vi "sensor de luz.vi"(8 "Error In":errorcluster, 10 "PIN Fotoresistencia":u8, 11 "LINX Resource":T1) -> (0 "Error Out":errorcluster, 2 "Miles de lumenes":dbl, 3 "LINX Resource 2":T1, 4 "Estado":string)   [LabVIEW 2014]
uses:
  <vilib>/MakerHub/LINX/Private/Type Defs/LINX Ref.ctl
  <vilib>/MakerHub/LINX/Private/Type Defs/Platform.ctl
  <vilib>/MakerHub/LINX/Private/Type Defs/Interface.ctl
  <vilib>/MakerHub/LINX/Private/Device/Type Defs/LINX Device Config.ctl
  <vilib>/MakerHub/LINX/Private/Device/Type Defs/TCP Config.ctl
  <vilib>/MakerHub/LINX/Private/Device/Type Defs/Channels.ctl
  <vilib>/MakerHub/LINX/Public/Peripherals/Analog/Analog Read 1 Chan.vi
  <vilib>/MakerHub/LINX/LMH-LINX.lvlib
  <vilib>/MakerHub/LINX/Private/Device/Device.lvlib
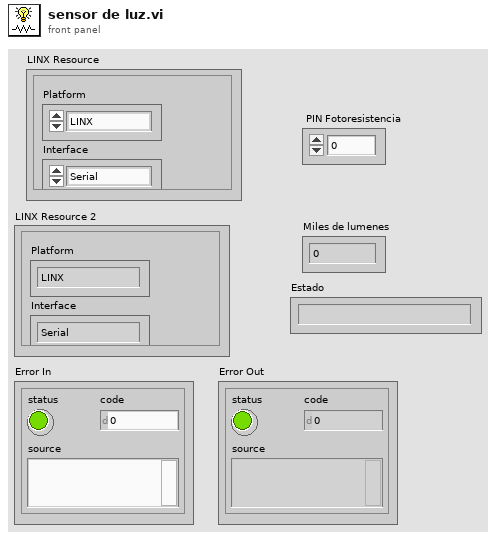
[diagram p1: front panel]
types:
  T1 = typedef "LMH-LINX.lvlib/LINX Ref.ctl" = cluster{"Platform":T2, "Interface":T3, "LINX Device Config":T4}
  T2 = typedef "LMH-LINX.lvlib/Platform.ctl" = enum16{"LINX", "myRIO"}
  T3 = typedef "LMH-LINX.lvlib/Interface.ctl" = enum16{"Serial", "TCP"}
  T4 = typedef "LMH-LINX.lvlib/Device.lvlib/LINX Device Config.ctl" = cluster{"Interface":T3, "COM Port":refnum<visa-resource-name>, "TCP Configuration":T5, "Device Family":u8, "Device ID":u8, "Device Name":string, "TCP Ref":refnum<k5>, "Channels":T6}
  T5 = typedef "LMH-LINX.lvlib/Device.lvlib/TCP Config.ctl" = cluster{"IP Address":string, "Port":u16}
  T6 = typedef "LMH-LINX.lvlib/Channels.ctl" = cluster{"DI":u8[], "DO":u8[], "AI":u8[], "AO":u8[], "PWM":u8[], "QE":u8[], "UART":u8[], "I2C 2":u8[], "SPI":u8[], "CAN":u8[], "Servo":u8[], "AI Ref (V)":dbl, "AO Ref (V)":dbl, "AO Resolution (Bits)":u8}
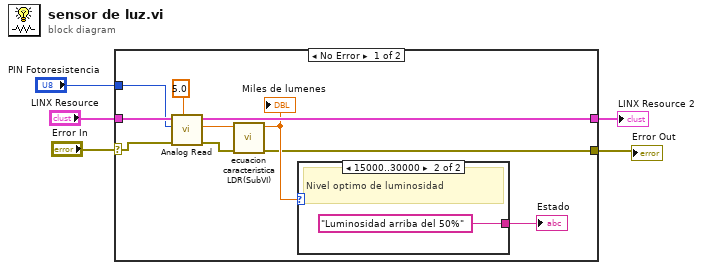
[diagram p0: block diagram]
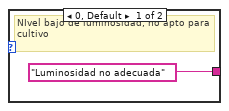
[diagram p2: hidden frame]
diagram:
  n1 = case shown="No Error" "Error In" {
    selector: "Error In" -> [w14 w18]
    tunnel: "LINX Resource" -> [w15 w19]
    tunnel: "PIN Fotoresistencia" -> [w12 _]
    tunnel: [w11 w19] -> w2
    tunnel: [w7 w18] -> w1
    frame No Error {
      n2 = call-poly <vilib>:"Analog Read.vi"("AI Range (V)"=5.0, "Error In"=w14, "Analog Channel"=w12, "LINX Resource"=w15) -> ("Error Out"=w8:errorcluster, "AI Value"=w13:dbl, "LINX Resource"=w11:T1)  [unwired: 4 in, 1 out]
      n3 = call "ecuacion caracteristica LDR(SubVI).vi"("Error In"=w8, "LDR"=w13) -> ("Error Out"=w7:errorcluster, "Miles de lumenes"=w9:dbl)  [unwired: 8 in]
      "Miles de lumenes" <- w9
      n4 = case shown="15000..30000" w9 {
        tunnel: ["Luminosidad no adecuada" "Luminosidad arriba del 50%"] -> w10
        frame 0, Default {
          # "NIvel bajo de luminosidad, no apto para cultivo"
        }
        frame 15000..30000 {
          # "Nivel optimo de luminosidad"
        }
      }
      "Estado" <- w10
    }
    frame Error {
    }
  }
  "Error Out" <- w1
  "LINX Resource 2" <- w2
